vi "move_3b.vi"(6 "Array in":i32[](array[numeric]), 9 "Array 3":i32[](array[numeric]), 10 "Array 5":i32[](array[numeric]), 11 "Enum in":enum16{"1", "2", "3"}(ring)) -> (1 "Array 6":i32[](array[numeric]), 2 "Enum 3":T1(ring), 3 "Enum out":T2(ring), 4 "Array 4":i32[](array[numeric]), 5 "Array out":i32[](array[numeric]))   [LabVIEW 2016]
uses:
  <vilib>/NXT/Block Support/NXT_OutputPort.ctl
  <vilib>/NXT/NXTIO Xnodes/NXTIONodeSubVIs/NXTStopMotors.vi
  <vilib>/NXT/NXTIO Xnodes/NXTIONodeSubVIs/NXTMotorRunDistance.vi
  <vilib>/NXT/NXTIO Xnodes/NXTIONodeSubVIs/LEGOMotorStatus.vi
  <vilib>/NXT/NXTIO Xnodes/NXTIONodeSubVIs/NXTMoveMotors.vi
  <vilib>/NXT/NXTIO Xnodes/NXTIONodeSubVIs/LEGOResetMotors.vi
  <vilib>/NXT/Subs/LVHSConnector.ctl
  <vilib>/NXT/NXTIO Xnodes/AddressXNode/NXTIOAddress.xnode
  <vilib>/NXT/NXTIO Xnodes/NXTIOXNode/NXTIO.xnode
  <vilib>/NXT/LegoClasses/BrickReference/BrickReference.lvclass
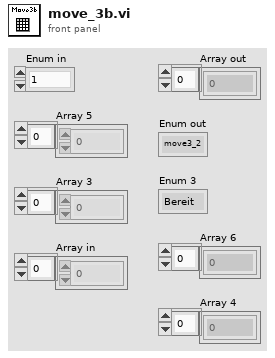
[diagram p1: front panel]
types:
  T1 = enum16{"Bereit", "Move 1", "Reference_pos", "Wait", "row1_check", "row2_check", "row3_check", "return", "move2", "move3", "move4", "move5", "end"}
  T2 = enum16{"move3_2", "move3_3", "move3_4", "move3_5"}
  T3 = enum16{"forward", "right", "mark", "pause", "up", "return", "end"}
  T4 = typedef "NXT_OutputPort.ctl" = u8
  T5 = cluster{"Output Port":T4, "Output Port 2":T4, "Output Port 3":T4}
  T6 = typedef "LVHSConnector.ctl" = refnum<class "BrickReference.lvclass">
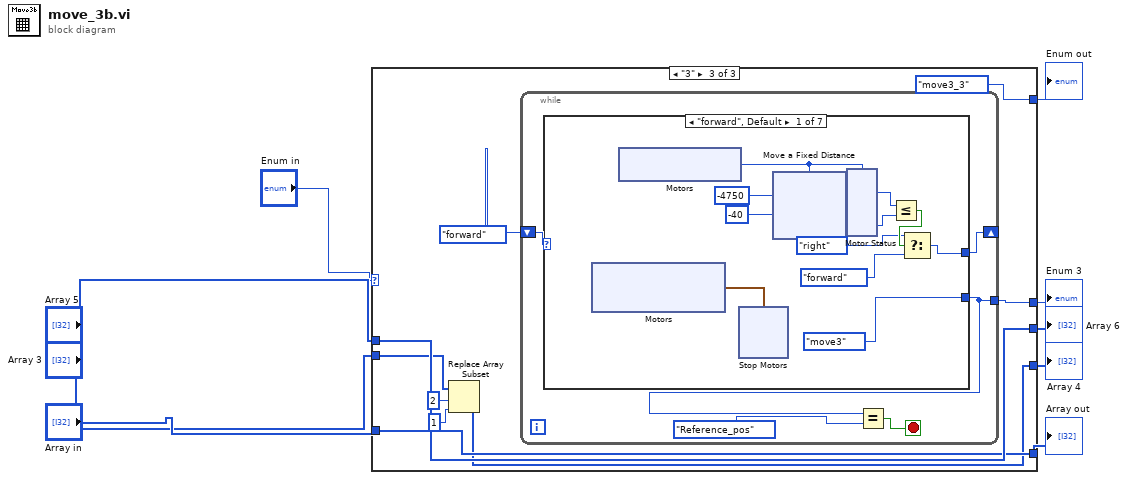
[diagram p0: block diagram]
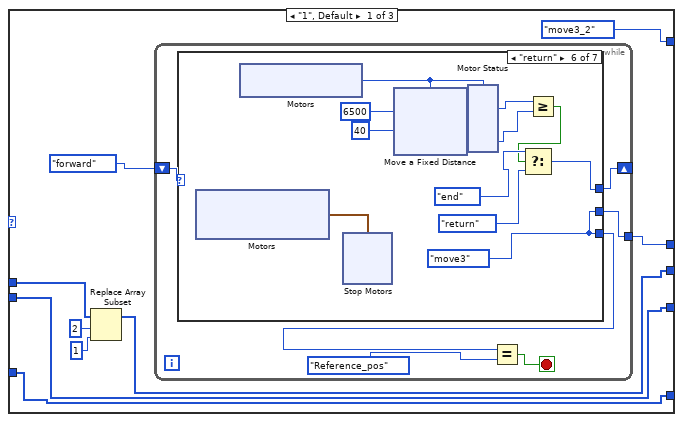
[diagram p2: hidden frame]
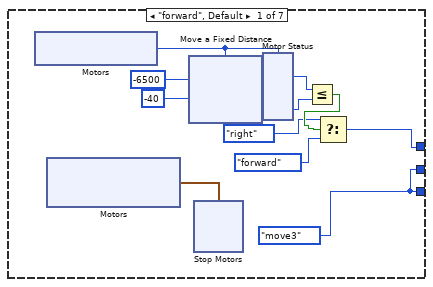
[diagram p3: hidden frame]
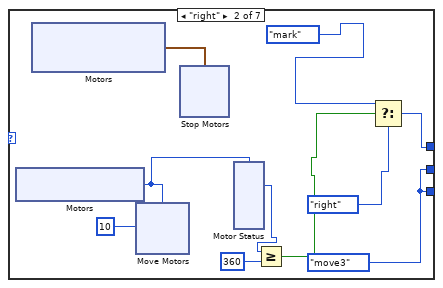
[diagram p4: hidden frame]
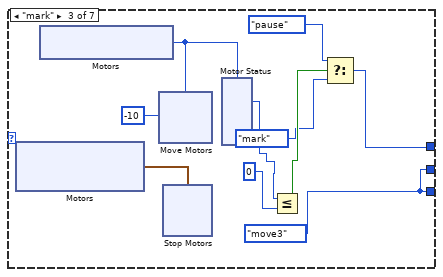
[diagram p5: hidden frame]
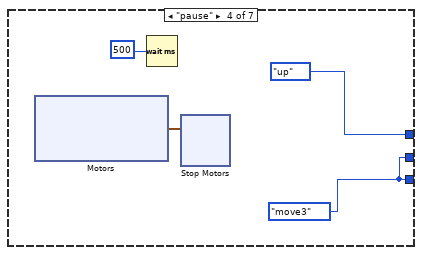
[diagram p6: hidden frame]
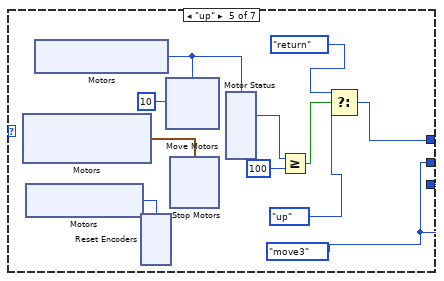
[diagram p7: hidden frame]
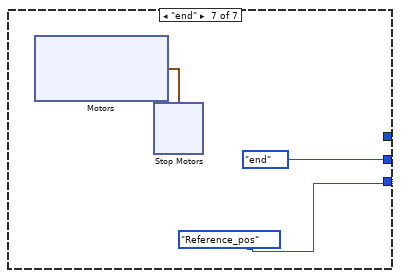
[diagram p8: hidden frame]
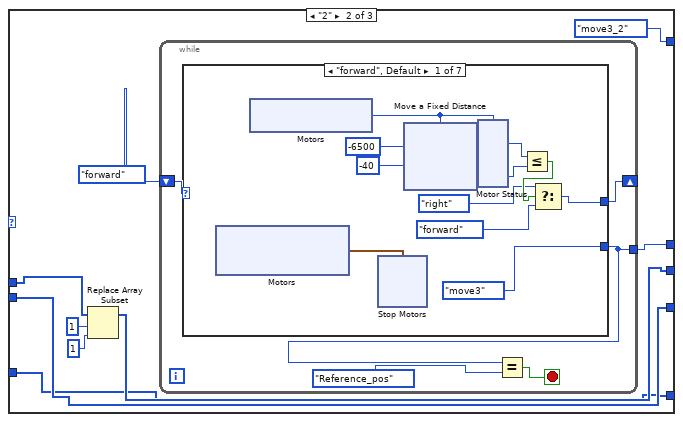
[diagram p9: hidden frame]
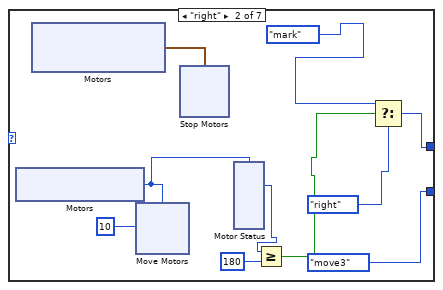
[diagram p10: hidden frame]
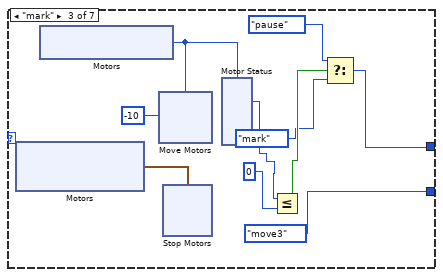
[diagram p11: hidden frame]
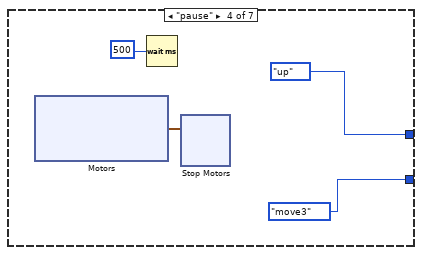
[diagram p12: hidden frame]
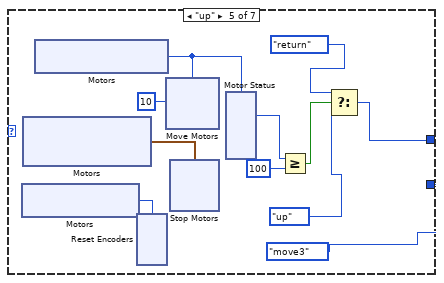
[diagram p13: hidden frame]
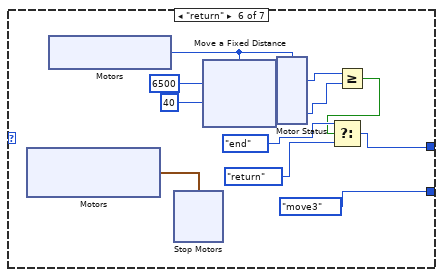
[diagram p14: hidden frame]
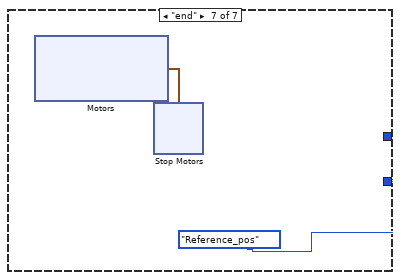
[diagram p15: hidden frame]
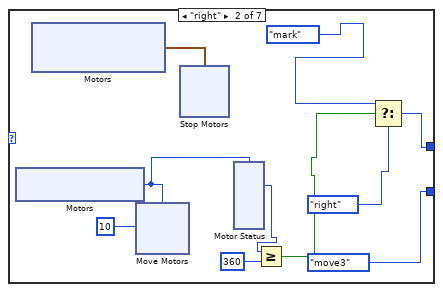
[diagram p16: hidden frame]
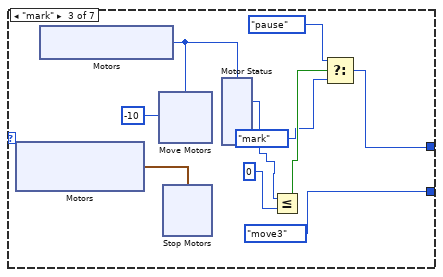
[diagram p17: hidden frame]
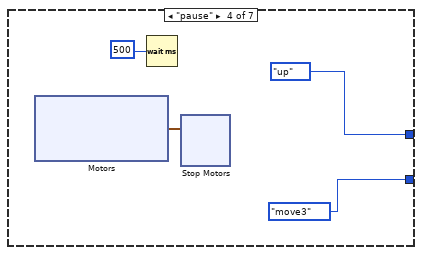
[diagram p18: hidden frame]
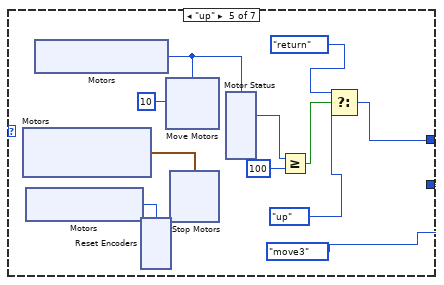
[diagram p19: hidden frame]
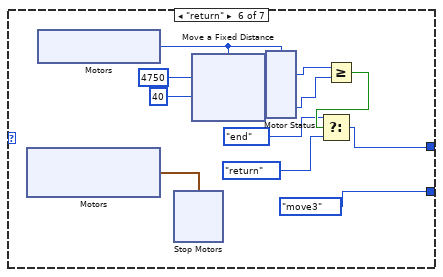
[diagram p20: hidden frame]
diagram:
  n1 = case shown="\"3\"" "Enum in" {
    tunnel: [w17 w225 w431] -> w1
    tunnel: [T2."move3_2" T2."move3_2" T2."move3_3"] -> w2
    tunnel: [w12 w220 w429] -> w4
    tunnel: "Array 5" -> [w13 w221 w429]
    tunnel: [w11 w219 w424] -> w6
    tunnel: "Array 3" -> [w11 w219 w425]
    tunnel: [w10 w218 w428] -> w8
    tunnel: "Array in" -> [w10 w218 w428]
    frame "1", Default {
      n2 = Replace Array Subset(array=w13, new element=1 ("new element/subarray"), index=2) -> (w12:i32[])
      n3 = while {
        shift-right: [w20] -> _
        shift-left: T3."forward" -> [w21]
        tunnel: [w19] -> w17
        stop <- w23 stop-if-true
        n4 = case shown="\"return\"" w21 {
          tunnel: [w25 w62 w94 T3."up" w137 w173 _] -> w20
          tunnel: [w34 w61 w93 w125 w136 w182 T1."Reference_pos"] -> w24
          tunnel: [w34 w61 w93 w125 w136 w182 T1."end"] -> w19
          frame "forward", Default {
            w29 = -6500 ("Distance 1")
            w34 = T1."move3"
            n5 = xnode "Motors"() -> ("Motor"=w31:T4)
            n6 = xnode "Motors"() -> ("Motor"=w35:cluster{"Port":T4, "Port":T4})
            n7 = xnode "Move a Fixed Distance"("Speed 1"=i8 -40, "Distance 1"=w29, "Motors"=w31) -> ("NXT/EV3"=w30:T6)  [unwired: 1 in]
            n8 = xnode "Stop Motors"("Motors"=w35) -> ()  [unwired: 1 in, 1 out]
            n9 = xnode "Motor Status"("Motors"=w31, "NXT/EV3"=w30) -> ("Position 1"=w32:i32)  [unwired: 2 out]
            n10 = Less Or Equal?(x=w32, y=w29) -> (x <= y?=w28:bool)
            n11 = Select(t=T3."right", s=w28, f=T3."forward") -> (s? t:f=w25:T3)
          }
          frame "right" {
            w61 = T1."move3"
            n12 = xnode "Motors"() -> ("Motor"=w70:T4)
            n13 = xnode "Motors"() -> ("Motor"=w69:cluster{"Port":T4, "Port":T4})
            n14 = xnode "Move Motors"("Power/Speed 1"=i8 10, "Motors"=w70) -> ()  [unwired: 1 in, 1 out]
            n15 = xnode "Stop Motors"("Motors"=w69) -> ()  [unwired: 1 in, 1 out]
            n16 = xnode "Motor Status"("Motors"=w70) -> ("Position 1"=w67:i32)  [unwired: 1 in, 2 out]
            n17 = Greater Or Equal?(x=w67, y=360) -> (x >= y?=w66:bool)
            n18 = Select(t=T3."mark", s=w66, f=T3."right") -> (s? t:f=w62:T3)
          }
          frame "mark" {
            w93 = T1."move3"
            n19 = xnode "Motors"() -> ("Motor"=w102:cluster{"Port":T4, "Port":T4})
            n20 = xnode "Motors"() -> ("Motor"=w100:T4)
            n21 = xnode "Move Motors"("Power/Speed 1"=i8 -10, "Motors"=w100) -> ()  [unwired: 1 in, 1 out]
            n22 = xnode "Stop Motors"("Motors"=w102) -> ()  [unwired: 1 in, 1 out]
            n23 = xnode "Motor Status"("Motors"=w100) -> ("Position 1"=w99:i32)  [unwired: 1 in, 2 out]
            n24 = Less Or Equal?(x=w99, y=0) -> (x <= y?=w97:bool)
            n25 = Select(t=T3."pause", s=w97, f=T3."mark") -> (s? t:f=w94:T3)
          }
          frame "pause" {
            w125 = T1."move3"
            n26 = xnode "Motors"() -> ("Motor"=w128:cluster{"Port":T4, "Port":T4, "Port":T4})
            n27 = Wait (ms)(milliseconds to wait=u32 500 ("millisecond timer value")) -> ()  [unwired: 1 out]
            n28 = xnode "Stop Motors"("Motors"=w128) -> ()  [unwired: 1 in, 1 out]
          }
          frame "up" {
            w136 = T1."move3"
            n29 = xnode "Motors"() -> ("Motor"=w144:cluster{"Port":T4, "Port":T4})
            n30 = xnode "Motors"() -> ("Motor"=w135:T4)
            n31 = xnode "Motors"() -> ("Motor"=w141:T4)
            n32 = xnode "Reset Encoders"("Motors"=w135) -> ()  [unwired: 1 in, 1 out]
            n33 = xnode "Move Motors"("Power/Speed 1"=i8 10, "Motors"=w141) -> ()  [unwired: 1 in, 1 out]
            n34 = xnode "Stop Motors"("Motors"=w144) -> ()  [unwired: 1 in, 1 out]
            n35 = xnode "Motor Status"("Motors"=w141) -> ("Position 1"=w142:i32)  [unwired: 1 in, 2 out]
            n36 = Greater Or Equal?(x=w142, y=100) -> (x >= y?=w143:bool)
            n37 = Select(t=T3."return", s=w143, f=T3."up") -> (s? t:f=w137:T3)
          }
          frame "return" {
            w177 = 6500 ("Distance 1")
            w182 = T1."move3"
            n38 = xnode "Motors"() -> ("Motor"=w183:cluster{"Port":T4, "Port":T4})
            n39 = xnode "Motors"() -> ("Motor"=w180:T4)
            n40 = xnode "Stop Motors"("Motors"=w183) -> ()  [unwired: 1 in, 1 out]
            n41 = xnode "Move a Fixed Distance"("Speed 1"=i8 40, "Distance 1"=w177, "Motors"=w180) -> ("NXT/EV3"=w179:T6)  [unwired: 1 in]
            n42 = xnode "Motor Status"("Motors"=w180, "NXT/EV3"=w179) -> ("Position 1"=w178:i32)  [unwired: 2 out]
            n43 = Greater Or Equal?(x=w178, y=w177) -> (x >= y?=w175:bool)
            n44 = Select(t=T3."end", s=w175, f=T3."return") -> (s? t:f=w173:T3)
          }
          frame "end" {
            n45 = xnode "Motors"() -> ("Motor"=w210:cluster{"Port":T4, "Port":T4, "Port":T4})
            n46 = xnode "Stop Motors"("Motors"=w210) -> ()  [unwired: 1 in, 1 out]
          }
        }
        n47 = Equal?(x=w24, y=T1."Reference_pos") -> (x = y?=w23:bool)
      }
    }
    frame "2" {
      n48 = Replace Array Subset(array=w221, new element=1 ("new element/subarray"), index=1) -> (w220:i32[])
      n49 = while {
        shift-right: [w227] -> _
        shift-left: T3."forward" -> [w228]
        tunnel: [w231] -> w225
        stop <- w230 stop-if-true
        n50 = case shown="\"forward\", Default" w228 {
          tunnel: [w232 w269 w301 T3."up" w343 w381 _] -> w227
          tunnel: [T1."move3" T1."move3" T1."move3" T1."move3" T1."move3" T1."move3" T1."Reference_pos"] -> w231
          frame "forward", Default {
            w236 = -6500 ("Distance 1")
            n51 = xnode "Motors"() -> ("Motor"=w242:cluster{"Port":T4, "Port":T4})
            n52 = xnode "Motors"() -> ("Motor"=w238:T4)
            n53 = xnode "Stop Motors"("Motors"=w242) -> ()  [unwired: 1 in, 1 out]
            n54 = xnode "Move a Fixed Distance"("Speed 1"=i8 -40, "Distance 1"=w236, "Motors"=w238) -> ("NXT/EV3"=w237:T6)  [unwired: 1 in]
            n55 = xnode "Motor Status"("Motors"=w238, "NXT/EV3"=w237) -> ("Position 1"=w239:i32)  [unwired: 2 out]
            n56 = Less Or Equal?(x=w239, y=w236) -> (x <= y?=w235:bool)
            n57 = Select(t=T3."right", s=w235, f=T3."forward") -> (s? t:f=w232:T3)
          }
          frame "right" {
            n58 = xnode "Motors"() -> ("Motor"=w277:T4)
            n59 = xnode "Motors"() -> ("Motor"=w276:cluster{"Port":T4, "Port":T4})
            n60 = xnode "Move Motors"("Power/Speed 1"=i8 10, "Motors"=w277) -> ()  [unwired: 1 in, 1 out]
            n61 = xnode "Stop Motors"("Motors"=w276) -> ()  [unwired: 1 in, 1 out]
            n62 = xnode "Motor Status"("Motors"=w277) -> ("Position 1"=w274:i32)  [unwired: 1 in, 2 out]
            n63 = Greater Or Equal?(x=w274, y=180) -> (x >= y?=w273:bool)
            n64 = Select(t=T3."mark", s=w273, f=T3."right") -> (s? t:f=w269:T3)
          }
          frame "mark" {
            n65 = xnode "Motors"() -> ("Motor"=w309:cluster{"Port":T4, "Port":T4})
            n66 = xnode "Motors"() -> ("Motor"=w307:T4)
            n67 = xnode "Move Motors"("Power/Speed 1"=i8 -10, "Motors"=w307) -> ()  [unwired: 1 in, 1 out]
            n68 = xnode "Stop Motors"("Motors"=w309) -> ()  [unwired: 1 in, 1 out]
            n69 = xnode "Motor Status"("Motors"=w307) -> ("Position 1"=w306:i32)  [unwired: 1 in, 2 out]
            n70 = Less Or Equal?(x=w306, y=0) -> (x <= y?=w304:bool)
            n71 = Select(t=T3."pause", s=w304, f=T3."mark") -> (s? t:f=w301:T3)
          }
          frame "pause" {
            n72 = xnode "Motors"() -> ("Motor"=w335:cluster{"Port":T4, "Port":T4, "Port":T4})
            n73 = Wait (ms)(milliseconds to wait=u32 500 ("millisecond timer value")) -> ()  [unwired: 1 out]
            n74 = xnode "Stop Motors"("Motors"=w335) -> ()  [unwired: 1 in, 1 out]
          }
          frame "up" {
            n75 = xnode "Motors"() -> ("Motor"=w342:T4)
            n76 = xnode "Motors"() -> ("Motor"=w350:cluster{"Port":T4, "Port":T4})
            n77 = xnode "Motors"() -> ("Motor"=w347:T4)
            n78 = xnode "Reset Encoders"("Motors"=w342) -> ()  [unwired: 1 in, 1 out]
            n79 = xnode "Move Motors"("Power/Speed 1"=i8 10, "Motors"=w347) -> ()  [unwired: 1 in, 1 out]
            n80 = xnode "Stop Motors"("Motors"=w350) -> ()  [unwired: 1 in, 1 out]
            n81 = xnode "Motor Status"("Motors"=w347) -> ("Position 1"=w348:i32)  [unwired: 1 in, 2 out]
            n82 = Greater Or Equal?(x=w348, y=100) -> (x >= y?=w349:bool)
            n83 = Select(t=T3."return", s=w349, f=T3."up") -> (s? t:f=w343:T3)
          }
          frame "return" {
            w384 = 6500 ("Distance 1")
            n84 = xnode "Motors"() -> ("Motor"=w389:cluster{"Port":T4, "Port":T4})
            n85 = xnode "Motors"() -> ("Motor"=w387:T4)
            n86 = xnode "Stop Motors"("Motors"=w389) -> ()  [unwired: 1 in, 1 out]
            n87 = xnode "Move a Fixed Distance"("Speed 1"=i8 40, "Distance 1"=w384, "Motors"=w387) -> ("NXT/EV3"=w386:T6)  [unwired: 1 in]
            n88 = xnode "Motor Status"("Motors"=w387, "NXT/EV3"=w386) -> ("Position 1"=w385:i32)  [unwired: 2 out]
            n89 = Greater Or Equal?(x=w385, y=w384) -> (x >= y?=w380:bool)
            n90 = Select(t=T3."end", s=w380, f=T3."return") -> (s? t:f=w381:T3)
          }
          frame "end" {
            n91 = xnode "Motors"() -> ("Motor"=w416:cluster{"Port":T4, "Port":T4, "Port":T4})
            n92 = xnode "Stop Motors"("Motors"=w416) -> ()  [unwired: 1 in, 1 out]
          }
        }
        n93 = Equal?(x=w231, y=T1."Reference_pos") -> (x = y?=w230:bool)
      }
    }
    frame "3" {
      n94 = Replace Array Subset(array=w425, new element=1 ("new element/subarray"), index=2) -> (w424:i32[])
      n95 = while {
        shift-right: [w433] -> _
        shift-left: T3."forward" -> [w434]
        tunnel: [w437] -> w431
        stop <- w436 stop-if-true
        n96 = case shown="\"forward\", Default" w434 {
          tunnel: [w438 w475 w507 T3."up" w549 w586 _] -> w433
          tunnel: [T1."move3" T1."move3" T1."move3" T1."move3" T1."move3" T1."move3" T1."Reference_pos"] -> w437
          frame "forward", Default {
            w442 = -4750 ("Distance 1")
            n97 = xnode "Motors"() -> ("Motor"=w448:cluster{"Port":T4, "Port":T4})
            n98 = xnode "Motors"() -> ("Motor"=w444:T4)
            n99 = xnode "Stop Motors"("Motors"=w448) -> ()  [unwired: 1 in, 1 out]
            n100 = xnode "Move a Fixed Distance"("Speed 1"=i8 -40, "Distance 1"=w442, "Motors"=w444) -> ("NXT/EV3"=w443:T6)  [unwired: 1 in]
            n101 = xnode "Motor Status"("Motors"=w444, "NXT/EV3"=w443) -> ("Position 1"=w445:i32)  [unwired: 2 out]
            n102 = Less Or Equal?(x=w445, y=w442) -> (x <= y?=w441:bool)
            n103 = Select(t=T3."right", s=w441, f=T3."forward") -> (s? t:f=w438:T3)
          }
          frame "right" {
            n104 = xnode "Motors"() -> ("Motor"=w483:T4)
            n105 = xnode "Motors"() -> ("Motor"=w482:cluster{"Port":T4, "Port":T4})
            n106 = xnode "Move Motors"("Power/Speed 1"=i8 10, "Motors"=w483) -> ()  [unwired: 1 in, 1 out]
            n107 = xnode "Stop Motors"("Motors"=w482) -> ()  [unwired: 1 in, 1 out]
            n108 = xnode "Motor Status"("Motors"=w483) -> ("Position 1"=w480:i32)  [unwired: 1 in, 2 out]
            n109 = Greater Or Equal?(x=w480, y=360) -> (x >= y?=w479:bool)
            n110 = Select(t=T3."mark", s=w479, f=T3."right") -> (s? t:f=w475:T3)
          }
          frame "mark" {
            n111 = xnode "Motors"() -> ("Motor"=w515:cluster{"Port":T4, "Port":T4})
            n112 = xnode "Motors"() -> ("Motor"=w513:T4)
            n113 = xnode "Move Motors"("Power/Speed 1"=i8 -10, "Motors"=w513) -> ()  [unwired: 1 in, 1 out]
            n114 = xnode "Stop Motors"("Motors"=w515) -> ()  [unwired: 1 in, 1 out]
            n115 = xnode "Motor Status"("Motors"=w513) -> ("Position 1"=w512:i32)  [unwired: 1 in, 2 out]
            n116 = Less Or Equal?(x=w512, y=0) -> (x <= y?=w510:bool)
            n117 = Select(t=T3."pause", s=w510, f=T3."mark") -> (s? t:f=w507:T3)
          }
          frame "pause" {
            n118 = xnode "Motors"() -> ("Motor"=w541:cluster{"Port":T4, "Port":T4, "Port":T4})
            n119 = Wait (ms)(milliseconds to wait=u32 500 ("millisecond timer value")) -> ()  [unwired: 1 out]
            n120 = xnode "Stop Motors"("Motors"=w541) -> ()  [unwired: 1 in, 1 out]
          }
          frame "up" {
            n121 = xnode "Motors"() -> ("Motor"=w556:cluster{"Port":T4, "Port":T4})
            n122 = xnode "Motors"() -> ("Motor"=w548:T4)
            n123 = xnode "Motors"() -> ("Motor"=w553:T4)
            n124 = xnode "Reset Encoders"("Motors"=w548) -> ()  [unwired: 1 in, 1 out]
            n125 = xnode "Move Motors"("Power/Speed 1"=i8 10, "Motors"=w553) -> ()  [unwired: 1 in, 1 out]
            n126 = xnode "Stop Motors"("Motors"=w556) -> ()  [unwired: 1 in, 1 out]
            n127 = xnode "Motor Status"("Motors"=w553) -> ("Position 1"=w554:i32)  [unwired: 1 in, 2 out]
            n128 = Greater Or Equal?(x=w554, y=100) -> (x >= y?=w555:bool)
            n129 = Select(t=T3."return", s=w555, f=T3."up") -> (s? t:f=w549:T3)
          }
          frame "return" {
            w590 = 4750 ("Distance 1")
            n130 = xnode "Motors"() -> ("Motor"=w595:cluster{"Port":T4, "Port":T4})
            n131 = xnode "Motors"() -> ("Motor"=w593:T4)
            n132 = xnode "Stop Motors"("Motors"=w595) -> ()  [unwired: 1 in, 1 out]
            n133 = xnode "Move a Fixed Distance"("Speed 1"=i8 40, "Distance 1"=w590, "Motors"=w593) -> ("NXT/EV3"=w592:T6)  [unwired: 1 in]
            n134 = xnode "Motor Status"("Motors"=w593, "NXT/EV3"=w592) -> ("Position 1"=w591:i32)  [unwired: 2 out]
            n135 = Greater Or Equal?(x=w591, y=w590) -> (x >= y?=w589:bool)
            n136 = Select(t=T3."end", s=w589, f=T3."return") -> (s? t:f=w586:T3)
          }
          frame "end" {
            n137 = xnode "Motors"() -> ("Motor"=w622:cluster{"Port":T4, "Port":T4, "Port":T4})
            n138 = xnode "Stop Motors"("Motors"=w622) -> ()  [unwired: 1 in, 1 out]
          }
        }
        n139 = Equal?(x=w437, y=T1."Reference_pos") -> (x = y?=w436:bool)
      }
    }
  }
  "Array out" <- w8
  "Array 4" <- w6
  "Array 6" <- w4
  "Enum out" <- w2
  "Enum 3" <- w1
